vi "AuMT8852B Change Register Enable.vi"(5 "Flags (all disabled)":T1, 7 "Set/Get (Set)":enum16{"Set", "Get"}(ring), 8 "error in (no error)":errorcluster, 10 "Value (-1)":i32=-1, 11 "VISA session":refnum<visa-resource-name>) -> (0 "error out":errorcluster, 2 "error code":i32, 3 "VISA session out":refnum<visa-resource-name>, 4 "Flags out":T1)   [LabVIEW 2017]
doc: "Anritsu MT8852B Bluetooth Tester\n\nThe bits in the Change Enable Register are the same as those in the Change Register. The two registers are bitwise AND'ed to determine whether to set the CHG bit in the Status Register.\n\nINPUTS\nSet/Get - whether the values are being written to or read from the instrument.\nFlags - individual values to assign to the register affecting the SCO connection status, USB status and AFH status.\nValue - integer value (0-255) to be written to the register. Leave this input unwired if you are using the Flags input.\n\nOUTPUTS\nFlags out - value of each bit in the register.\nValue out - integer value (0-255) of the register."
panel:
  out "Value out":i32
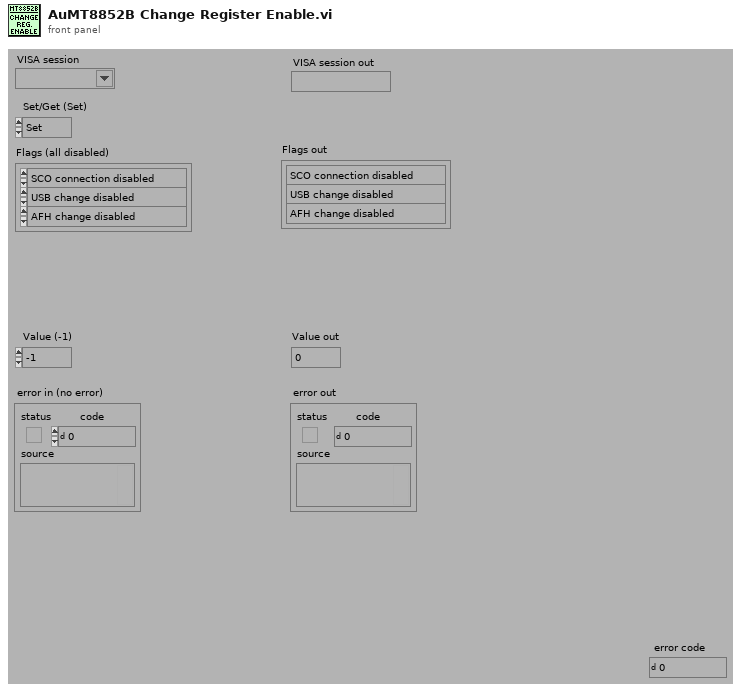
[diagram p1: front panel]
types:
  T1 = cluster{"SCO Connection":enum16{"SCO connection disabled", "SCO connection enabled"}, "USB Change":enum16{"USB change disabled", "USB change enabled"}, "AFH Change":enum16{"AFH change disabled", "AFH change enabled"}}
  T2 = enum16{"Simulate", "Range check", "Cache", "Query instrument status"}
  T3 = enum16{"SCO connection disabled", "SCO connection enabled"}
  T4 = enum16{"USB change disabled", "USB change enabled"}
  T5 = enum16{"AFH change disabled", "AFH change enabled"}
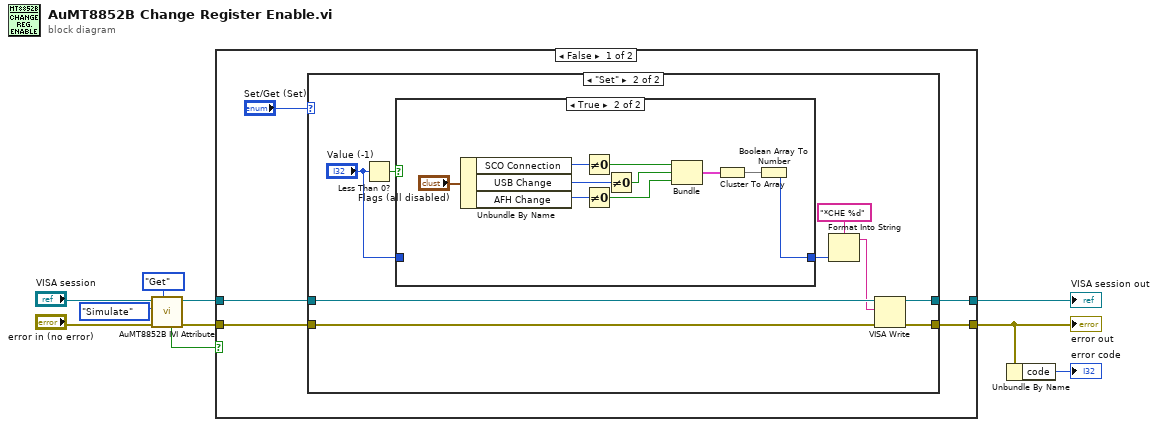
[diagram p0: block diagram]
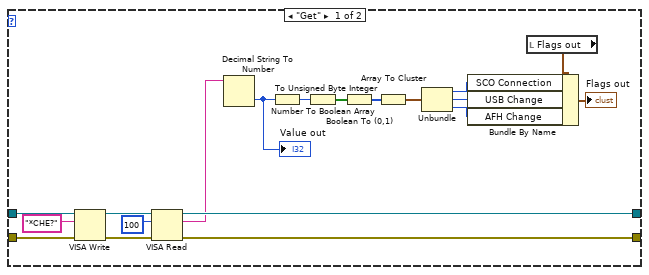
[diagram p2: hidden frame]
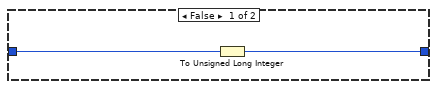
[diagram p3: hidden frame]
diagram:
  n1 = call <instrlib>:"AuMT8852B IVI Attribute.vi"("Set/Get (Set)"=enum16{"Set", "Get"}."Get", "error in (no error)"="error in (no error)", "Flag (Simulate)"=T2."Simulate", "VISA session"="VISA session") -> ("error out"=w6:errorcluster, "VISA session out"=w7:refnum<visa-resource-name>, "Value out"=w3:bool)  [unwired: 5 in]
  n2 = case shown="False" w3 {
    tunnel: [w12 w56] -> w1
    tunnel: [w13 w57] -> w8
    tunnel: w7 -> [w15 w57]
    tunnel: w6 -> [w14 w56]
    frame False {
      n3 = case shown="\"Set\"" "Set/Get (Set)" {
        tunnel: w15 -> [w34 w43]
        tunnel: w14 -> [w33 w42]
        tunnel: [w29 w39] -> w13
        tunnel: [w28 w38] -> w12
        frame "Get" {
          n4 = VISA Write(VISA resource name=w34, write buffer="*CHE?" ("write buffer (\"\")"), error in (no error)=w33) -> (VISA resource name out=w31:refnum<visa-resource-name>, error out=w30:errorcluster)  [unwired: 1 out]
          n5 = VISA Read(VISA resource name=w31, byte count=u32 100 ("byte count (0)"), error in (no error)=w30) -> (VISA resource name out=w29:refnum<visa-resource-name>, read buffer=w26:string, error out=w28:errorcluster)  [unwired: 1 out]
          n6 = Decimal String To Number(string=w26) -> (number=w20:i32)  [unwired: 2 in, 1 out]
          "Value out" <- w20
          n7 = To Unsigned Byte Integer(number=w20) -> (unsigned 8bit integer=w21:u8)
          n8 = Number To Boolean Array(number=w21) -> (Boolean array=w22:bool[])
          n9 = Boolean To (0,1)(Boolean=w22) -> (0, 1=w23:i16[])
          n10 = Array To Cluster(array=w23) -> (cluster=w24:cluster{"[0]":i16, "[1]":i16, "[2]":i16})
          n11 = Unbundle(w24) -> ("[0]"=w19:i16, "[1]"=w18:i16, "[2]"=w17:i16)
          n12 = local read "Flags out"() -> (w25:T1)
          n13 = Bundle By Name(cluster=w25, "SCO Connection"=w19, "USB Change"=w18, "AFH Change"=w17) -> (→"Flags out":T1)
        }
        frame "Set" {
          n14 = Less Than 0?(x="Value (-1)") -> (x < 0?=w36:bool)
          n15 = case shown="True" w36 {
            tunnel: [w44 w55] -> w40
            tunnel: "Value (-1)" -> [w45 _]
            frame False {
              n16 = To Unsigned Long Integer(number=w45) -> (unsigned 32bit integer=w44:u32)
            }
            frame True {
              n17 = Unbundle By Name("Flags (all disabled)") -> ("SCO Connection"=w53:T3, "USB Change"=w51:T4, "AFH Change"=w49:T5)
              n18 = Not Equal To 0?(x=w53) -> (x != 0?=w52:bool)
              n19 = Not Equal To 0?(x=w49) -> (x != 0?=w48:bool)
              n20 = Not Equal To 0?(x=w51) -> (x != 0?=w50:bool)
              n21 = Bundle(w52, w50, w48) -> (w47:cluster{bool, bool, bool})  [unwired: 1 in]
              n22 = Cluster To Array(cluster=w47) -> (array=w46:bool[])
              n23 = Boolean Array To Number(Boolean array=w46) -> (number=w55:u32)
            }
          }
          n24 = Format Into String(format string="*CHE %d" ("Format String"), w40) -> (resulting string=w37:string)  [unwired: 2 in, 1 out]
          n25 = VISA Write(VISA resource name=w43, write buffer=w37, error in (no error)=w42) -> (VISA resource name out=w39:refnum<visa-resource-name>, error out=w38:errorcluster)  [unwired: 1 out]
        }
      }
    }
    frame True {
    }
  }
  "error out" <- w1
  "VISA session out" <- w8
  n26 = Unbundle By Name(w1) -> ("code"=→"error code":i32)
